vi "wdt_analog_multiplewrites.vi"() -> ()   [LabVIEW 2019]
uses:
  <vilib>/Analysis/NI_AALBase.lvlib
panel:
  out "t0":timestamp=timestamp(3655728074.5497446 s since 1904-01-01)
  out "Error Out":errorcluster
  in  "TDMS File":path=path "C:/Python/projects/nitdms/tests/tdms_files/wdt_analog_multiplewrites.tdms"
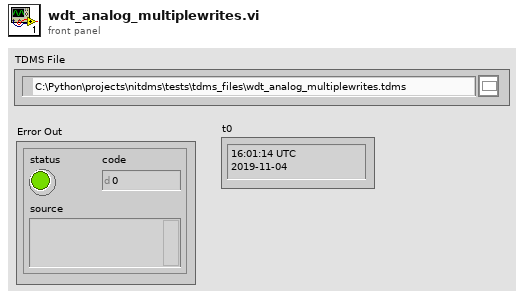
[diagram p1: front panel]
types:
  T1 = enum16{"open", "open or create", "create or replace", "create", "open (read-only)"}
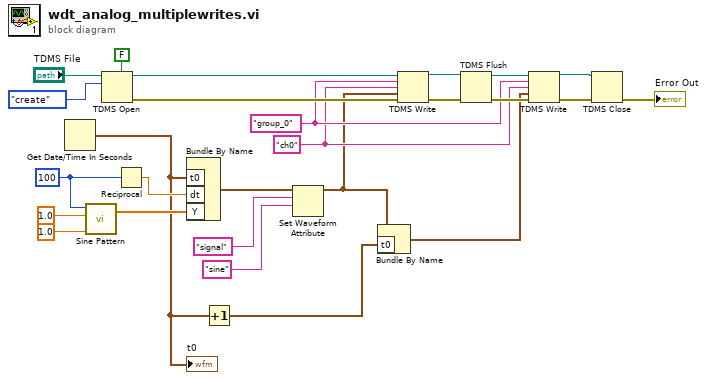
[diagram p0: block diagram]
diagram:
  w5 = "group_0" ("name")
  w4 = "ch0" ("name")
  w20 = 100 ("samples")
  n1 = Get Date/Time In Seconds() -> (seconds since 1Jan1904=w12:timestamp)
  "t0" <- w12
  n2 = call <vilib>:"Sine Pattern.vi"("cycles"=1.0, "amplitude"=1.0, "samples"=w20) -> ("Sinusoidal Pattern"=w21:dbl[])  [unwired: 1 in, 1 out]
  n3 = TDMS Open(5:FALSE ("create index file? (T)"), 10:T1."create" ("operation (0:open)"), 11:"TDMS File") -> (0:w16:errorcluster, 3:w15:refnum<k34>)  [unwired: 4 in]
  n4 = Reciprocal(x=w20) -> (1/x=w19:dbl)
  n5 = Bundle By Name("t0"=w12, "dt"=w19, "Y"=w21) -> (w18:waveform(dbl))  [unwired: 1 in]
  n6 = Increment(x=w12) -> (x+1=w2:timestamp)
  n7 = Set Waveform Attribute(5:"sine" ("name"), 6:"signal" ("name"), 7:w18) -> (3:w3:waveform(dbl))  [unwired: 1 in, 2 out]
  n8 = Bundle By Name(cluster=w3, "t0"=w2) -> (w1:waveform(dbl))
  n9 = TDMS Write(0:w15, 5:w5, 7:w4, 9:w3, 11:w16) -> (4:w10:refnum<k34>, 15:w11:errorcluster)  [unwired: 1 in, 2 out]
  n10 = TDMS Flush(4:w11, 7:w10) -> (0:w9:errorcluster, 3:w7:refnum<k34>)
  n11 = TDMS Write(0:w7, 5:w5, 7:w4, 9:w1, 11:w9) -> (4:w6:refnum<k34>, 15:w8:errorcluster)  [unwired: 1 in, 2 out]
  n12 = TDMS Close(8:w8, 11:w6) -> (0:→"Error Out":errorcluster)  [unwired: 1 out]
